vi "Func-엑셀 데이터를 그래프로 출력.vi"() -> ()   [LabVIEW 2015] (continued)
110.16\n110.18\n110.19\n110.21\n110.23\n110.24\n110.26\n110.28\n110.29\n110.31\n110.33\n110.34\n110.36\n110.38\n110.39\n110.41\n110.43\n110.44\n110.46\n110.48\n110.49\n110.51\n110.53\n110.54\n110.56\n110.58\n110.59\n110.61\n110.63\n110.64\n110.66\n110.68\n110.69\n110.71\n110.73\n110.75\n110.76\n110.78\n110.79\n110.81\n110.83\n110.84\n110.86\n110.88\n110.89\n110.91\n110.93\n110.94\n110.96\n110.98\n110.99\n111.01\n111.03\n111.04\n111.06\n111.08\n111.09\n111.11\n111.13\n111.14\n111.16\n111.18\n111.19\n111.21\n111.23\n111.24\n111.26\n111.28\n111.29\n111.31\n111.33\n111.34\n111.36\n111.38\n111.39\n111.41\n111.43\n111.45\n111.46\n111.48\n111.49\n111.51\n111.53\n111.55\n111.56\n111.58\n111.59\n111.61\n111.63\n111.64\n111.66\n111.68\n111.69\n111.71\n111.73\n111.74\n111.76\n111.78\n111.8\n111.81\n111.83\n111.84\n111.86\n111.88\n111.9\n111.91\n111.93\n111.95\n111.96\n111.98\n111.99\n112.01\n112.03\n112.04\n112.06\n112.08\n112.09\n112.11\n112.13\n112.15\n112.16\n112.18\n112.19\n112.21\n112.23\n112.25\n112.26\n112.28\n112.29\n112.31\n112.33\n112.34\n112.36\n112.38\n112.39\n112.41\n112.43\n112.44\n112.46\n112.48\n112.5\n112.51\n112.53\n112.54\n112.56\n112.58\n112.6\n112.61\n112.63\n112.64\n112.66\n112.68\n112.69\n112.71\n112.73\n112.74\n112.76\n112.78\n112.79\n112.81\n112.83\n112.84\n112.86\n112.88\n112.89\n112.91\n112.93\n112.95\n112.96\n112.98\n113\n113.01\n113.03\n113.04\n113.06\n113.08\n113.09\n113.11\n113.13\n113.14\n113.16\n113.18\n113.19\n113.21\n113.23\n113.24\n113.26\n113.28\n113.29\n113.31\n113.33\n113.34\n113.36\n113.38\n113.39\n113.41\n113.43\n113.44\n113.46\n113.48\n113.5\n113.51\n113.53\n113.54\n113.56\n113.58\n113.59\n113.61\n113.63\n113.64\n113.66\n113.68\n113.69\n113.71\n113.73\n113.74\n113.76\n113.78\n113.79\n113.81\n113.83\n113.84\n113.86\n113.88\n113.89\n113.91\n113.93\n113.94\n113.96\n113.98\n113.99\n114.01\n114.03\n114.04\n114.06\n114.08\n114.09\n114.11\n114.13\n114.14\n114.16\n114.18\n114.19\n114.21\n114.23\n114.24\n114.26\n114.28\n114.29\n114.31\n114.33\n114.34\n114.36\n114.38\n114.39\n114.41\n114.43\n114.44\n114.46\n114.48\n114.49\n114.51\n114.53\n114.54\n114.56\n114.58\n114.59\n114.61\n114.63\n114.64\n114.66\n114.68\n114.7\n114.71\n114.73\n114.74\n114.76\n114.78\n114.79\n114.81\n114.83\n114.84\n114.86\n114.88\n114.9\n114.91\n114.93\n114.94\n114.96\n114.98\n115\n115.01\n115.03\n115.04\n115.06\n115.08\n115.09\n115.11\n115.13\n115.14\n115.16\n115.18\n115.19\n115.21\n115.23\n115.25\n115.26\n115.28\n115.29\n115.31\n115.33\n115.35\n115.36\n115.38\n115.39\n115.41\n115.43\n115.44\n115.46\n115.48\n115.5\n115.51\n115.53\n115.54\n115.56\n115.58\n115.59\n115.61\n115.63\n115.64\n115.66\n115.68\n115.7\n115.71\n115.73\n115.74\n115.76\n115.78\n115.79\n115.81\n115.83\n115.84\n115.86\n115.88\n115.89\n115.91\n115.93\n115.94\n115.96\n115.98\n115.99\n116.01\n116.03\n116.04\n116.06\n116.08\n116.09\n116.11\n116.13\n116.15\n116.16\n116.18\n116.19\n116.21\n116.23\n116.24\n116.26\n116.28\n116.29\n116.31\n116.33\n116.34\n116.36\n116.38\n116.39\n116.41\n116.43\n116.44\n116.46\n116.48\n116.49\n116.51\n116.53\n116.54\n116.56\n116.58\n116.6\n116.61\n116.63\n116.64\n116.66\n116.68\n116.69\n116.71\n116.73\n116.74\n116.76\n116.78\n116.79\n116.81\n116.83\n116.84\n116.86\n116.88\n116.89\n116.91\n116.93\n116.94\n116.96\n116.98\n116.99\n117.01\n117.03\n117.04\n117.06\n117.08\n117.09\n117.11\n117.13\n117.14\n117.16\n117.18\n117.19\n117.21\n117.23\n117.24\n117.26\n117.28\n117.29\n117.31\n117.33\n117.34\n117.36\n117.38\n117.39\n117.41\n117.43\n117.44\n117.46\n117.48\n117.49\n117.51\n117.53\n117.54\n117.56\n117.58\n117.59\n117.61\n117.63\n117.65\n117.66\n117.68\n117.69\n117.71\n117.73\n117.74\n117.76\n117.78\n117.79\n117.81\n117.83\n117.84\n117.86\n117.88\n117.89\n117.91\n117.93\n117.94\n117.96\n117.98\n118\n118.01\n118.03\n118.04\n118.06\n118.08\n118.1\n118.11\n118.13\n118.14\n118.16\n118.18\n118.19\n118.21\n118.23\n118.24\n118.26\n118.28\n118.29\n118.31\n118.33\n118.35\n118.36\n118.38\n118.39\n118.41\n118.43\n118.45\n118.46\n118.48\n118.49\n118.51\n118.53\n118.54\n118.56\n118.58\n118.59\n118.61\n118.63\n118.64\n118.66\n118.68\n118.69\n118.71\n118.73\n118.74\n118.76\n118.78\n118.79\n118.81\n118.83\n118.84\n118.86\n118.88\n118.89\n118.91\n118.93\n118.94\n118.96\n118.98\n118.99\n119.01\n119.03\n119.04\n119.06\n119.08\n119.09\n119.11\n119.13\n119.14\n119.16\n119.18\n119.19\n119.21\n119.23\n119.25\n119.26\n119.28\n119.29\n119.31\n119.33\n119.34\n119.36\n119.38\n119.39\n119.41\n119.43\n119.44\n119.46\n119.48\n119.49\n119.51\n119.53\n119.54\n119.56\n119.58\n119.59\n119.61\n119.63\n119.64\n119.66\n119.68\n119.69\n119.71\n119.73\n119.74\n119.76\n119.78\n119.79\n119.81\n119.83\n119.84\n119.86\n119.88\n119.89\n119.91\n119.93\n119.94\n119.96\n119.98\n119.99\n120.01\n120.03\n120.05\n120.06\n120.08\n120.09\n120.11\n120.13\n120.14\n120.16\n120.18\n120.19\n120.21\n120.23\n120.24\n120.26\n120.28\n120.29\n120.31\n120.33\n120.34\n120.36\n120.38\n120.39\n120.41\n120.43\n120.44\n120.46\n120.48\n120.49\n120.51\n120.53\n120.54\n120.56\n120.58\n120.59\n120.61\n120.63\n120.64\n120.66\n120.68\n120.69\n120.71\n120.73\n120.74\n120.76\n120.78\n120.79\n120.81\n120.83\n120.84\n120.86\n120.88\n120.89\n120.91\n120.93\n120.94\n120.96\n120.98\n120.99\n121.01\n121.03\n121.04\n121.06\n121.08\n121.1\n121.11\n121.13\n121.14\n121.16\n121.18\n121.2\n121.21\n121.23\n121.24\n121.26\n121.28\n121.29\n121.31\n121.33\n121.34\n121.36\n121.38\n121.39\n121.41\n121.43\n121.45\n121.46\n121.48\n121.49\n121.51\n121.53\n121.55\n121.56\n121.58\n121.6\n121.61\n121.63\n121.64\n121.66\n121.68\n121.69\n121.71\n121.73\n121.74\n121.76\n121.78\n121.79\n121.81\n121.83\n121.84\n121.86\n121.88\n121.9\n121.91\n121.93\n121.94\n121.96\n121.98\n121.99\n122.01\n122.03\n122.04\n122.06\n122.08\n122.09\n122.11\n122.13\n122.14\n122.16\n122.18\n122.19\n122.21\n122.23\n122.25\n122.26\n122.28\n122.29\n122.31\n122.33\n122.34\n122.36\n122.38\n122.39\n122.41\n122.43\n122.44\n122.46\n122.48\n122.49\n122.51\n122.53\n122.54\n122.56\n122.58\n122.59\n122.61\n122.63\n122.64\n122.66\n122.68\n122.69\n122.71\n122.73\n122.74\n122.76\n122.78\n122.79\n122.81\n122.83\n122.84\n122.86\n122.88\n122.89\n122.91\n122.93\n122.94\n122.96\n122.98\n122.99\n123.01\n123.03\n123.04\n123.06\n123.08\n123.09\n123.11\n123.13\n123.14\n123.16\n123.18\n123.19\n123.21\n123.23\n123.24\n123.26\n123.28\n123.29\n123.31\n123.33\n123.34\n123.36\n123.38\n123.39\n123.41\n123.43\n123.44\n123.46\n123.48\n123.49\n123.51\n123.53\n123.54\n123.56\n123.58\n123.59\n123.61\n123.63\n123.64\n123.66\n123.68\n123.69\n123.71\n123.73\n123.74\n123.76\n123.78\n123.79\n123.81\n123.83\n123.84\n123.86\n123.88\n123.89\n123.91\n123.93\n123.94\n123.96\n123.98\n123.99\n124.01\n124.03\n124.04\n124.06\n124.08\n124.1\n124.11\n124.13\n124.14\n124.16\n124.18\n124.19\n124.21\n124.23\n124.24\n124.26\n124.28\n124.3\n124.31\n124.33\n124.34\n124.36\n124.38\n124.39\n124.41\n124.43\n124.44\n124.46\n124.48\n124.49\n124.51\n124.53\n124.55\n124.56\n124.58\n124.59\n124.61\n124.63\n124.65\n124.66\n124.68\n124.69\n124.71\n124.73\n124.74\n124.76\n124.78\n124.8\n124.81\n124.83\n124.84\n124.86\n124.88\n124.89\n124.91\n124.93\n124.94\n124.96\n124.98\n124.99\n125.01\n125.03\n125.04\n125.06\n125.08\n125.09\n125.11\n125.13\n125.14\n125.16\n125.18\n125.19\n125.21\n125.23\n125.25\n125.26\n125.28\n125.29\n125.31\n125.33\n125.34\n125.36\n125.38\n125.39\n125.41\n125.43\n125.44\n125.46\n125.48\n125.49\n125.51\n125.53\n125.54\n125.56\n125.58\n125.59\n125.61\n125.63\n125.64\n125.66\n125.68\n125.69\n125.71\n125.73\n125.74\n125.76\n125.78\n125.79\n125.81\n125.83\n125.84\n125.86\n125.88\n125.89\n125.91\n125.93\n125.94\n125.96\n125.98\n125.99\n126.01\n126.03\n126.04\n126.06\n126.08\n126.09\n126.11\n126.13\n126.14\n126.16\n126.18\n126.19\n126.21\n126.23\n126.24\n126.26\n126.28\n126.29\n126.31\n126.33\n126.34\n126.36\n126.38\n126.39\n126.41\n126.43\n126.44\n126.46\n126.48\n126.49\n126.51\n126.53\n126.54\n126.56\n126.58\n126.59\n126.61\n126.63\n126.64\n126.66\n126.68\n126.69\n126.71\n126.73\n126.74\n126.76\n126.78\n126.79\n126.81\n126.83\n126.84\n126.86\n126.88\n126.89\n126.91\n126.93\n126.94\n126.96\n126.98\n126.99\n127.01\n127.03\n127.05\n127.06\n127.08\n127.09\n127.11\n127.13\n127.14\n127.16\n127.18\n127.2\n127.21\n127.23\n127.24\n127.26\n127.28\n127.3\n127.31\n127.33\n127.34\n127.36\n127.38\n127.4\n127.41\n127.43\n127.44\n127.46\n127.48\n127.49\n127.51\n127.53\n127.54\n127.56\n127.58\n127.59\n127.61\n127.63\n127.65\n127.66\n127.68\n127.69\n127.71\n127.73\n127.75\n127.76\n127.78\n127.79\n127.81\n127.83\n127.84\n127.86\n127.88\n127.9\n127.91\n127.93\n127.94\n127.96\n127.98\n128\n128.01\n128.03\n128.04\n128.06\n128.08\n128.1\n128.11\n128.13\n128.14\n128.16\n128.18\n128.19\n128.21\n128.23\n128.24\n128.26\n128.28\n128.29\n128.31\n128.33\n128.34\n128.36\n128.38\n128.39\n128.41\n128.43\n128.44\n128.46\n128.48\n128.49\n128.51\n128.53\n128.54\n128.56\n128.58\n128.59\n128.61\n128.63\n128.64\n128.66\n128.68\n128.69\n128.71\n128.73\n128.74\n128.76\n128.78\n128.79\n128.81\n128.83\n128.84\n128.86\n128.88\n128.89\n128.91\n128.93\n128.94\n128.96\n128.98\n128.99\n129.01\n129.03\n129.04\n129.06\n129.08\n129.09\n129.11\n129.13\n129.14\n129.16\n129.18\n129.19\n129.21\n129.23\n129.24\n129.26\n129.28\n129.29\n129.31\n129.33\n129.34\n129.36\n129.38\n129.39\n129.41\n129.43\n129.44\n129.46\n129.48\n129.49\n129.51\n129.53\n129.54\n129.56\n129.58\n129.59\n129.61\n129.63\n129.64\n129.66\n129.68\n129.69\n129.71\n129.73\n129.74\n129.76\n129.78\n129.79\n129.81\n129.83\n129.85\n129.86\n129.88\n129.89\n129.91\n129.93\n129.94\n129.96\n129.98\n129.99\n130.01\n130.03\n130.04\n130.06\n130.08\n130.09\n130.11\n130.13\n130.15\n130.16\n130.18\n130.19\n130.21\n130.23\n130.24\n130.26\n130.28\n130.3\n130.31\n130.33\n130.34\n130.36\n130.38\n130.4\n130.41\n130.43\n130.44\n130.46\n130.48\n130.5\n130.51\n130.53\n130.54\n130.56\n130.58\n130.59\n130.61\n130.63\n130.64\n130.66\n130.68\n130.69\n130.71\n130.73\n130.75\n130.76\n130.78\n130.79\n130.81\n130.83\n130.85\n130.86\n130.88\n130.89\n130.91\n130.93\n130.94\n130.96\n130.98\n130.99\n131.01\n131.03\n131.04\n131.06\n131.08\n131.09\n131.11\n131.13\n131.14\n131.16\n131.18\n131.19\n131.21\n131.23\n131.24\n131.26\n131.28\n131.3\n131.31\n131.33\n131.35\n131.36\n131.38\n131.39\n131.41\n131.43\n131.44\n131.46\n131.48\n131.49\n131.51\n131.53\n131.54\n131.56\n131.58\n131.59\n131.61\n131.63\n131.64\n131.66\n131.68\n131.69\n131.71\n131.73\n131.74\n131.76\n131.78\n131.79\n131.81\n131.83\n131.84\n131.86\n131.88\n131.89\n131.91\n131.93\n131.94\n131.96\n131.98\n131.99\n132.01\n132.03\n132.04\n132.06\n132.08\n132.09\n132.11\n132.13\n132.14\n132.16\n132.18\n132.19\n132.21\n132.23\n132.24\n132.26\n132.28\n132.29\n132.31\n132.33\n132.34\n132.36\n132.38\n132.39\n132.41\n132.43\n132.44\n132.46\n132.48\n132.49\n132.51\n132.53\n132.54\n132.56\n132.58\n132.59\n132.61\n132.63\n132.64\n132.66\n132.68\n132.69\n132.71\n132.73\n132.74\n132.76\n132.78\n132.8\n132.81\n132.83\n132.84\n132.86\n132.88\n132.89\n132.91\n132.93\n132.94\n132.96\n132.98\n132.99\n133.01\n133.03\n133.04\n133.06\n133.08\n133.09\n133.11\n133.13\n133.14\n133.16\n133.18\n133.19\n133.21\n133.23\n133.25\n133.26\n133.28\n133.29\n133.31\n133.33\n133.34\n133.36\n133.38\n133.4\n133.41\n133.43\n133.44\n133.46\n133.48\n133.5\n133.51\n133.53\n133.54\n133.56\n133.58\n133.59\n133.61\n133.63\n133.64\n133.66\n133.68\n133.69\n133.71\n133.73\n133.74\n133.76\n133.78\n133.79\n133.81\n133.83\n133.85\n133.86\n133.88\n133.89\n133.91\n133.93\n133.95\n133.96\n133.98\n133.99\n134.01\n134.03\n134.04\n134.06\n134.08\n134.09\n134.11\n134.13\n134.14\n134.16\n134.18\n134.19\n134.21\n134.23\n134.24\n134.26\n134.28\n134.29\n134.31\n134.33\n134.34\n134.36\n134.38\n134.39\n134.41\n134.43\n134.44\n134.46\n134.48\n134.49\n134.51\n134.53\n134.54\n134.56\n134.58\n134.59\n134.61\n134.63\n134.65\n134.66\n134.68\n134.69\n134.71\n134.73\n134.74\n134.76\n134.78\n134.79\n134.81\n134.83\n134.84\n134.86\n134.88\n134.89\n134.91\n134.93\n134.94\n134.96\n134.98\n134.99\n135.01\n135.03\n135.04\n135.06\n135.08\n135.09\n135.11\n135.13\n135.14\n135.16\n135.18\n135.19\n135.21\n135.23\n135.24\n135.26\n135.28\n135.29\n135.31\n135.33\n135.34\n135.36\n135.38\n135.39\n135.41\n135.43\n135.44\n135.46\n135.48\n135.49\n135.51\n135.53\n135.54\n135.56\n135.58\n135.59\n135.61\n135.63\n135.64\n135.66\n135.68\n135.69\n135.71\n135.73\n135.74\n135.76\n135.78\n135.79\n135.81\n135.83\n135.84\n135.86\n135.88\n135.9\n135.91\n135.93\n135.94\n135.96\n135.98\n136\n136.01\n136.03\n136.04\n136.06\n136.08\n136.09\n136.11\n136.13\n136.14\n136.16\n136.18\n136.19\n136.21\n136.23\n136.24\n136.26\n136.28\n136.29\n136.31\n136.33\n136.34\n136.36\n136.38\n136.39\n136.41\n136.43\n136.44\n136.46\n136.48\n136.49\n136.51\n136.53\n136.54\n136.56\n136.58\n136.59\n136.61\n136.63\n136.64\n136.66\n136.68\n136.7\n136.71\n136.73\n136.74\n136.76\n136.78\n136.79\n136.81\n136.83\n136.84\n136.86\n136.88\n136.89\n136.91\n136.93\n136.95\n136.96\n136.98\n136.99\n137.01\n137.03\n137.05\n137.06\n137.08\n137.09\n137.11\n137.13\n137.14\n137.16\n137.18\n137.2\n137.21\n137.23\n137.24\n137.26\n137.28\n137.3\n137.31\n137.33\n137.34\n137.36\n137.38\n137.39\n137.41\n137.43\n137.45\n137.46\n137.48\n137.49\n137.51\n137.53\n137.54\n137.56\n137.58\n137.59\n137.61\n137.63\n137.64\n137.66\n137.68\n137.69\n137.71\n137.73\n137.74\n137.76\n137.78\n137.79\n137.81\n137.83\n137.84\n137.86\n137.88\n137.89\n137.91\n137.93\n137.94\n137.96\n137.98\n137.99\n138.01\n138.03\n138.04\n138.06\n138.08\n138.09\n138.11\n138.13\n138.14\n138.16\n138.18\n138.19\n138.21\n138.23\n138.24\n138.26\n138.28\n138.29\n138.31\n138.33\n138.34\n138.36\n138.38\n138.39\n138.41\n138.43\n138.44\n138.46\n138.48\n138.49\n138.51\n138.53\n138.55\n138.56\n138.58\n138.59\n138.61\n138.63\n138.64\n138.66\n138.68\n138.69\n138.71\n138.73\n138.74\n138.76\n138.78\n138.79\n138.81\n138.83\n138.84\n138.86\n138.88\n138.89\n138.91\n138.93\n138.94\n138.96\n138.98\n139\n139.01\n139.03\n139.04\n139.06\n139.08\n139.09\n139.11\n139.13\n139.14\n139.16\n139.18\n139.19\n139.21\n139.23\n139.24\n139.26\n139.28\n139.29\n139.31\n139.33\n139.34\n139.36\n139.38\n139.39\n139.41\n139.43\n139.44\n139.46\n139.48\n139.49\n139.51\n139.53\n139.54\n139.56\n139.58\n139.59\n139.61\n139.63\n139.64\n139.66\n139.68\n139.7\n139.71\n139.73\n139.74\n139.76\n139.78\n139.8\n139.81\n139.83\n139.84\n139.86\n139.88\n139.89\n139.91\n139.93\n139.95\n139.96\n139.98\n139.99\n140.01\n140.03\n140.05\n140.06\n140.08\n140.1\n140.11\n140.13\n140.15\n140.16\n140.18\n140.19\n140.21\n140.23\n140.24\n140.26\n140.28\n140.29\n140.31\n140.33\n140.34\n140.36\n140.38\n140.4\n140.41\n140.43\n140.44\n140.46\n140.48\n140.5\n140.51\n140.53\n140.55\n140.56\n140.58\n140.59\n140.61\n140.63\n140.64\n140.66\n140.68\n140.69\n140.71\n140.73\n140.74\n140.76\n140.78\n140.79\n140.81\n140.83\n140.84\n140.86\n140.88\n140.89\n140.91\n140.93\n140.94\n140.96\n140.98\n140.99\n141.01\n141.03\n141.04\n141.06\n141.08\n141.09\n141.11\n141.13\n141.14\n141.16\n141.18\n141.19\n141.21\n141.23\n141.24\n141.26\n141.28\n141.29\n141.31\n141.33\n141.34\n141.36\n141.38\n141.39\n141.41\n141.43\n141.44\n141.46\n141.48\n141.49\n141.51\n141.53\n141.54\n141.56\n141.58\n141.59\n141.61\n141.63\n141.64\n141.66\n141.68\n141.69\n141.71\n141.73\n141.74\n141.76\n141.78\n141.79\n141.81\n141.83\n141.84\n141.86\n141.88\n141.89\n141.91\n141.93\n141.94\n141.96\n141.98\n141.99\n142.01\n142.03\n142.04\n142.06\n142.08\n142.09\n142.11\n142.13\n142.14\n142.16\n142.18\n142.19\n142.21\n142.23\n142.24\n142.26\n142.28\n142.29\n142.31\n142.33\n142.34\n142.36\n142.38\n142.39\n142.41\n142.43\n142.44\n142.46\n142.48\n142.49\n142.51\n142.53\n142.54\n142.56\n142.58\n142.59\n142.61\n142.63\n142.64\n142.66\n142.68\n142.69\n142.71\n142.73\n142.74\n142.76\n142.78\n142.79\n142.81\n142.83\n142.84\n142.86\n142.88\n142.9\n142.91\n142.93\n142.94\n142.96\n142.98\n142.99\n143.01\n143.03\n143.05\n143.06\n143.08\n143.09\n143.11\n143.13\n143.15\n143.16\n143.18\n143.19\n143.21\n143.23\n143.25\n143.26\n143.28\n143.29\n143.31\n143.33\n143.34\n143.36\n143.38\n143.39\n143.41\n143.43\n143.44\n143.46\n143.48\n143.49\n143.51\n143.53\n143.54\n143.56\n143.58\n143.59\n143.61\n143.63\n143.64\n143.66\n143.68\n143.69\n143.71\n143.73\n143.74\n143.76\n143.78\n143.79\n143.81\n143.83\n143.84\n143.86\n143.88\n143.89\n143.91\n143.93\n143.94\n143.96\n143.98\n143.99\n144.01\n144.03\n144.04\n144.06\n144.08\n144.1\n144.11\n144.13\n144.14\n144.16\n144.18\n144.19\n144.21\n144.23\n144.24\n144.26\n144.28\n144.29\n144.31\n144.33\n144.34\n144.36\n144.38\n144.39\n144.41\n144.43\n144.44\n144.46\n144.48\n144.49\n144.51\n144.53\n144.54\n144.56\n144.58\n144.59\n144.61\n144.63\n144.64\n144.66\n144.68\n144.69\n144.71\n144.73\n144.74\n144.76\n144.78\n144.79\n144.81\n144.83\n144.84\n144.86\n144.88\n144.89\n144.91\n144.93\n144.94\n144.96\n144.98\n144.99\n145.01\n145.03\n145.04\n145.06\n145.08\n145.09\n145.11\n145.13\n145.14\n145.16\n145.18\n145.19\n145.21\n145.23\n145.24\n161.47\n161.64\n161.81\n161.97\n162.14\n162.31\n162.47\n162.64\n162.81\n162.97\n163.14\n163.31\n163.47\n163.64\n163.81\n163.97\n164.14\n164.31\n164.47\n164.64\n164.81\n164.97\n165.15\n165.31\n165.48\n165.65\n165.81\n165.98\n166.15\n166.31\n166.48\n166.65\n166.81\n166.98\n167.15\n167.31\n167.48\n167.65\n167.81\n167.98\n168.15\n168.31\n168.48\n168.65\n168.81\n168.98\n169.15\n169.31\n169.48\n169.65\n169.81\n169.98\n170.15\n170.31\n170.48\n170.65\n170.82\n170.98\n171.15\n171.31\n171.48\n171.65\n171.81\n171.98\n172.15\n172.31\n172.48\n172.65\n172.81\n172.98\n173.15\n173.32\n173.49\n173.66\n173.82\n173.99\n174.16\n174.32\n174.49\n174.66\n174.82\n174.99\n175.16\n175.32\n175.49\n175.66\n175.82\n175.99\n176.16\n176.32\n176.5\n176.67\n176.83\n177\n177.16\n177.33\n177.5\n177.66\n177.83\n178\n178.16\n178.33\n178.5\n178.66\n178.83\n179\n179.16\n179.33\n179.5\n179.66\n179.83\n180\n180.16\n180.33\n180.5\n180.66\n180.83\n181\n181.16\n181.33\n181.5\n181.66\n181.83\n182\n182.16\n182.33\n182.5\n182.66\n182.83\n183\n183.16\n183.33\n183.5\n183.66\n183.83\n184\n184.16\n184.33\n184.5\n184.66\n184.83\n185\n185.16\n185.33\n185.5\n185.66\n185.83\n186\n186.16\n186.33\n186.5\n186.67\n186.84\n187.01\n187.17\n187.34\n187.51\n187.67\n187.84\n188.01\n188.17\n188.34\n188.51\n188.67\n188.84\n189.01\n189.17\n189.34\n189.51\n189.67\n189.85\n190.01\n190.18\n190.35\n190.51\n190.68\n190.85\n191.01\n191.18\n191.35\n191.51\n191.68\n191.85\n192.01\n192.18\n192.35\n192.52\n192.68\n192.85\n193.01\n193.18\n193.35\n193.51\n193.68\n193.85\n194.01\n194.18\n194.35\n194.51\n194.68\n194.85\n195.01\n195.18\n195.35\n195.51\n195.68\n195.85\n196.01\n196.18\n196.35\n196.51\n196.68\n196.85\n197.01\n197.18\n197.35\n197.51\n197.68\n197.85\n198.02\n198.19\n198.36\n198.52\n198.69\n198.86\n199.02\n199.19\n199.36\n199.52\n199.69\n199.86\n200.02\n200.19\n200.36\n200.52\n200.69\n200.86\n201.02\n201.19\n201.36\n201.52\n201.69\n201.86\n202.02\n202.19\n202.36\n202.52\n202.69\n202.86\n203.02\n203.19\n203.36\n203.52\n203.69\n203.86\n204.02\n204.19\n204.36\n204.51\n204.51\n204.53\n204.55\n204.56\n204.58\n204.59\n204.61\n204.63\n204.65\n204.66\n204.68\n204.69\n204.71\n204.73\n204.74\n204.76\n204.78\n204.79\n204.81\n204.83\n204.84\n204.86\n204.88\n204.9\n204.91\n204.93\n204.94\n204.96\n204.98\n205\n205.01\n205.03\n205.04\n205.06\n205.08\n205.09\n205.11\n205.13\n205.15\n205.16\n205.18\n205.19\n205.21\n205.23\n205.24\n205.26\n205.28\n205.29\n205.31\n205.33\n205.34\n205.36\n205.38\n205.39\n205.41\n205.43\n205.44\n205.46\n205.48\n205.49\n205.51\n205.53\n205.54\n205.56\n205.58\n205.6\n205.61\n205.63\n205.64\n205.66\n205.68\n205.69\n205.71\n205.73\n205.74\n205.76\n205.78\n205.79\n205.81\n205.83\n205.84\n205.86\n205.88\n205.89\n205.91\n205.93\n205.94\n205.96\n205.98\n205.99\n206.01\n206.03\n206.04\n206.06\n206.08\n206.09\n206.11\n206.13\n206.14\n206.16\n206.18\n206.19\n206.21\n206.23\n206.24\n206.26\n206.28\n206.29\n206.31\n206.33\n206.34\n206.36\n206.38\n206.39\n206.41\n206.43\n206.44\n206.46\n206.48\n206.49\n206.51\n206.53\n206.54\n206.56\n206.58\n206.59\n206.61\n206.63\n206.64\n206.66\n206.68\n206.69\n206.71\n206.73\n206.74\n206.76\n206.78\n206.79\n206.81\n206.83\n206.84\n206.86\n206.88\n206.89\n206.91\n206.93\n206.94\n206.96
